vi "3D Shape Test Bench.vi"() -> ()   [LabVIEW 2017]
uses:
  <vilib>/picture/3D Picture Control/NI_3D Picture Control.lvlib
  <vilib>/robotics/Kinematics/NI_Kinematics.lvlib
  Controls/Room Dimensions.ctl
  <vilib>/userdefined/High Color/IMAQdx.ctl
  <vilib>/vision/Image Controls.llb/IMAQ Image.ctl
  <vilib>/vision/Avi.llb/IMAQ AVI2 Refnum.ctl
  Controls/Position.ctl
  Controls/Orientation.ctl
  Controls/Rigid Body Info.ctl
  Controls/Frame Grabber Data.ctl
  Controls/Dimensions.ctl
  Controls/Recording Settings.ctl
  Controls/Operator.ctl
  Controls/Operator Settings.ctl
  Controls/Refnums.ctl
  Controls/Patient Settings.ctl
panel:
  in  "Dimensions":T1={"Probe Dimensions"={"Probe Width"=0.0, "Probe Depth"=1.0, "Probe Height"=0.0}, "Room Dimensions"={"Room Width"=0.0, "Room Depth"=0.0, "Room Height"=0.0}}
  in  "Frame Grabber Data In":T3={"Camera Session"="", "Frame"="remote image 0000000019B07D24", "AVI Refnum"=refnum, "Codecs"=["Cinepak Codec by Radius", "Intel IYUV codec", "Microsoft Video 1", "FF Video Codec 1 (FFV1) (NI Vision)", "Motion JPEG (NI Vision)", "Y800 Uncompressed Grey Scale (NI Vision)", "YUV 4:2:0 Planar (NI Vision)"], "Frame number"=0, "Tracking File Refnum"=refnum, "Tick Count"=0, "Probe Object"=refnum, "Playback Probe Data"=[], "Rigid Body"={"Position"={"x (mm)"=0.0, "y (mm)"=0.0, "z (mm)"=0.0}, "Orientation"={"Pitch (rad)"=0.0, "Yaw (rad)"=0.0, "Roll (rad)"=0.0}, "Quaternion"={"qx"=0.0, "qy"=0.0, "qz"=0.0, "qw"=0.0}, "Tracked?"=FALSE}, "Total no frames playback"=0, "Video FPS"=0.0, "Camera connected?"=FALSE, "Scene"=refnum, "Cropped Frame"=refnum, "Tracker FPS"=0.0, "Crop ROI"=[], "Presentation Values"=[], "Elapsed time (ms)"=0, "Camera frames playback"=0, "Refnums"={"Live Refnum"=refnum, "Record Refnum"=refnum, "Playback Refnum"=refnum, "Frame Slider Refnum"=refnum, "Pause Refnum"=refnum, "Home Refnum"=refnum, "Set Crop Refnum"=refnum, "Clear Crop Refnum"=refnum, "stop refnum"=refnum, "Playback Rate Refnum"=refnum, "Presentation Refnum"=refnum, "Crop Time Frame Slider Refnum"=refnum, "Cancel Save Refnum"=refnum, "Reverse Playback Refnum"=refnum, "Recording Settings Refnum"=refnum, "Continuous Playback Refnum"=refnum, "Annotation Refnum"=refnum, "Export All Refnum"=refnum, "Export List Refnum"=refnum, "Fill List Refnum"=refnum, "Save Crop Refnum"=refnum, "Skip Forward Refnum"=refnum, "Skip Backward Refnum"=refnum, "Single Annotation Refnum"=refnum, "Load Video Refnum"=refnum, "Set Start Refnum"=refnum, "Set End Refnum"=refnum, "Add to List Refnum"=refnum, "List of Annotations Refnum"=refnum, "Camera Frame Refnum"=refnum, "Load Image Refnum"=refnum, "Saving Refnum"=refnum}, "Dimensions"={"Probe Dimensions"={"Probe Width"=0.0, "Probe Depth"=1.0, "Probe Height"=0.0}, "Room Dimensions"={"Room Width"=0.0, "Room Depth"=0.0, "Room Height"=0.0}}, "Playback Data As Strings"=[], "Cropped Tracking File Refnum"=refnum, "Cropped AVI Refnum"=refnum, "Header"=[], "Total euclidian distance"=0.0}
  out "Error Out":errorcluster={"status"=TRUE, "code"=1088, "source"="Property Node (arg 2) in NI_3D Picture Control.lvlib:Create Box.vi->Create 3D Shapes.vi->3D Shape Test Bench.vi"}
  in  "Error In":errorcluster
  in  "Initial Probe Position":cluster{"X":sgl, "Y":sgl, "Z":sgl}
  in  "Orientation":cluster{"X":sgl, "Y":sgl, "Z":sgl}
  in  "Stop Button":bool
  out "Scene":refnum<vi>(3d-picture)
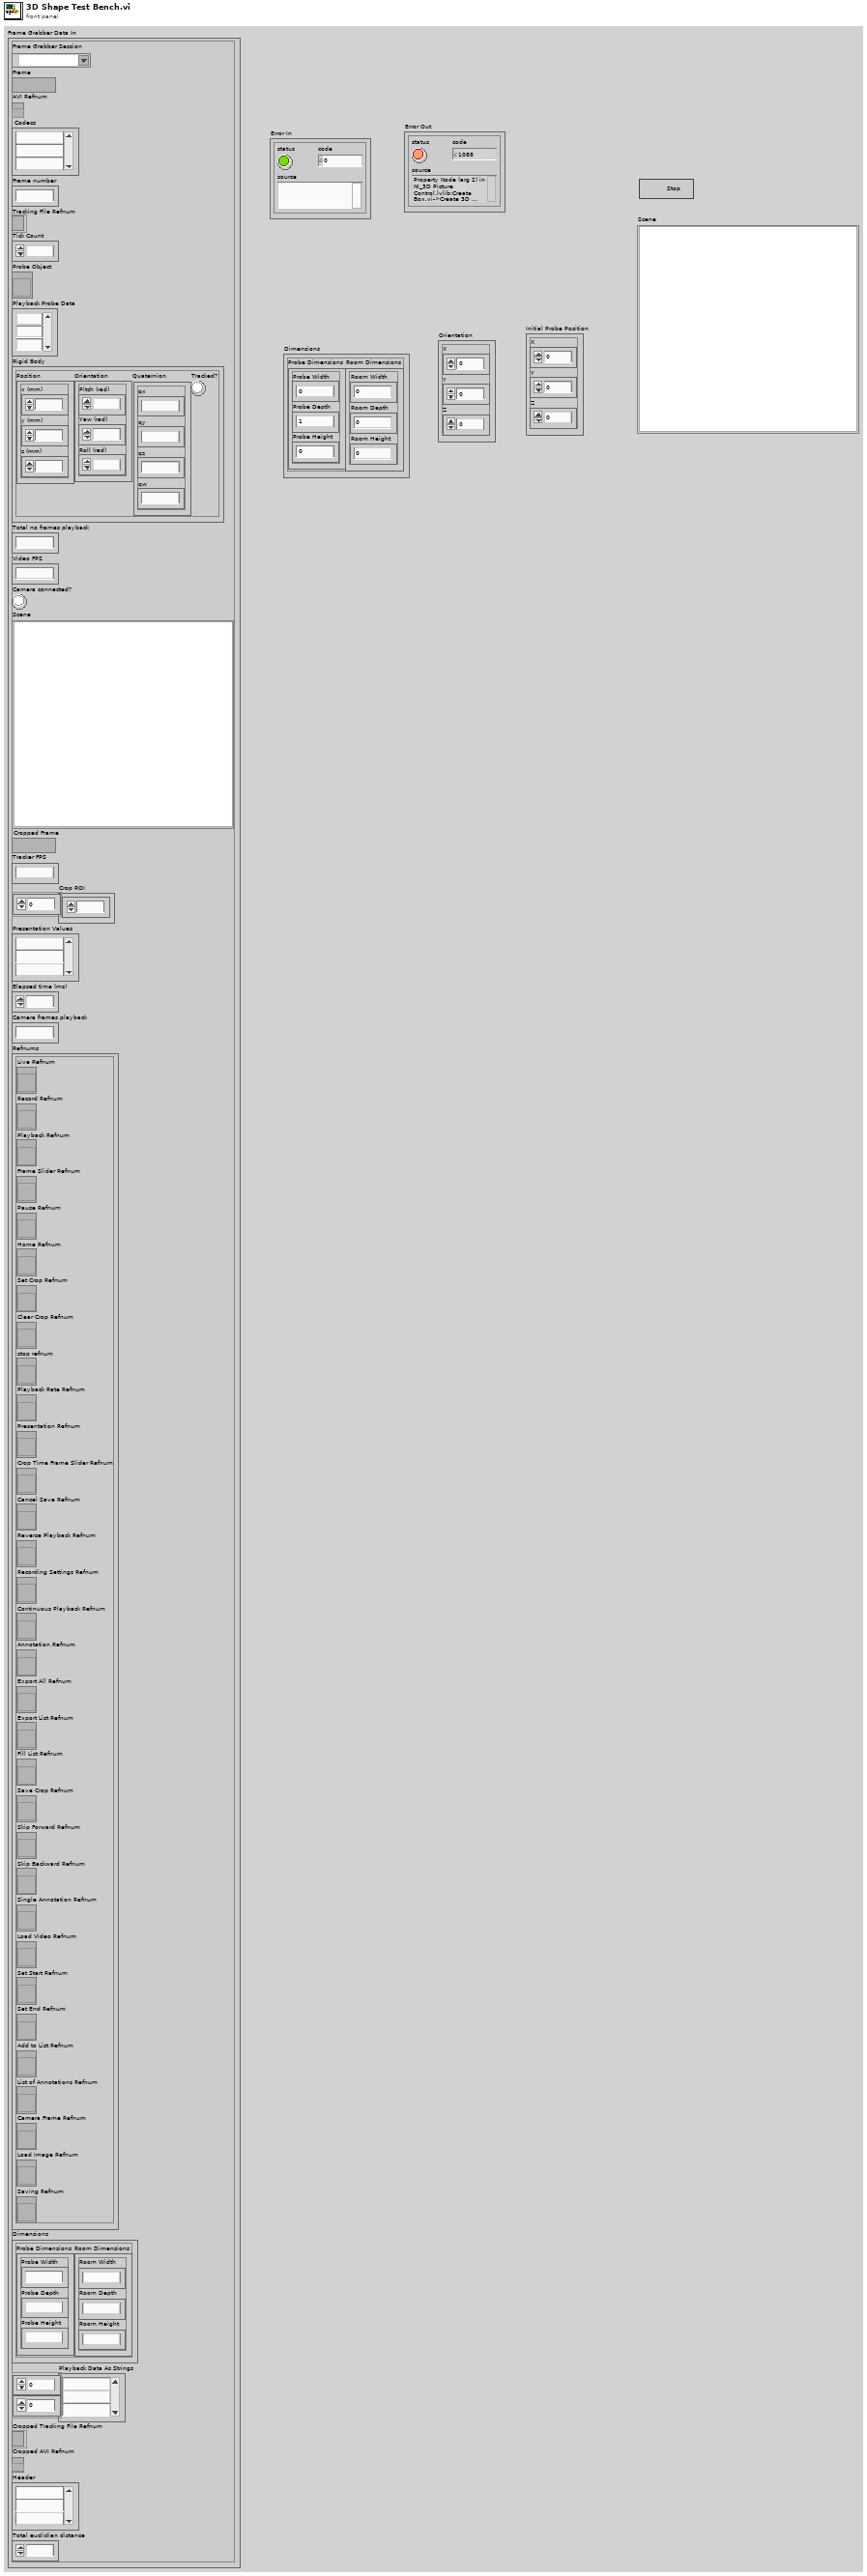
[diagram p1: front panel]
types:
  T1 = typedef "Dimensions.ctl" = cluster{"Probe Dimensions":cluster{"Probe Width":sgl, "Probe Depth":sgl, "Probe Height":sgl}, "Room Dimensions":T2}
  T2 = typedef "Room Dimensions.ctl" = cluster{"Room Width":dbl, "Room Depth":dbl, "Room Height":dbl}
  T3 = typedef "Frame Grabber Data.ctl" = cluster{"Camera Session":T4, "Frame":T5, "AVI Refnum":T6, "Codecs":string[], "Frame number":u32, "Tracking File Refnum":refnum<file>, "Tick Count":u32, "Probe Object":refnum<vi>, "Playback Probe Data":dbl[][], "Rigid Body":T7, "Total no frames playback":i32, "Video FPS":dbl, "Camera connected?":bool, "Scene":refnum<vi>, "Cropped Frame":T5, "Tracker FPS":dbl, "Crop ROI":i32[], "Presentation Values":string[], "Elapsed time (ms)":u32, "Camera frames playback":u32, "Refnums":T10, "Dimensions":T1, "Playback Data As Strings":string[][], "Cropped Tracking File Refnum":refnum<file>, "Cropped AVI Refnum":T6, "Header":string[], "Total euclidian distance":dbl}
  T4 = typedef "IMAQdx.ctl" = refnum<k21>
  T5 = typedef "IMAQ Image.ctl" = refnum<image>
  T6 = typedef "IMAQ AVI2 Refnum.ctl" = refnum<k20>
  T7 = typedef "Rigid Body Info.ctl" = cluster{"Position":T8, "Orientation":T9, "Quaternion":cluster{"qx":sgl, "qy":sgl, "qz":sgl, "qw":sgl}, "Tracked?":bool}
  T8 = typedef "Position.ctl" = cluster{"x (mm)":sgl, "y (mm)":sgl, "z (mm)":sgl}
  T9 = typedef "Orientation.ctl" = cluster{"Pitch (rad)":sgl, "Yaw (rad)":sgl, "Roll (rad)":sgl}
  T10 = typedef "Refnums.ctl" = cluster{"Live Refnum":refnum<vi>, "Record Refnum":refnum<vi>, "Playback Refnum":refnum<vi>, "Frame Slider Refnum":refnum<vi>, "Pause Refnum":refnum<vi>, "Home Refnum":refnum<vi>, "Set Crop Refnum":refnum<vi>, "Clear Crop Refnum":refnum<vi>, "stop refnum":refnum<vi>, "Playback Rate Refnum":refnum<vi>, "Presentation Refnum":refnum<vi>, "Crop Time Frame Slider Refnum":refnum<vi>, "Cancel Save Refnum":refnum<vi>, "Reverse Playback Refnum":refnum<vi>, "Recording Settings Refnum":refnum<vi>, "Continuous Playback Refnum":refnum<vi>, "Annotation Refnum":refnum<vi>, "Export All Refnum":refnum<vi>, "Export List Refnum":refnum<vi>, "Fill List Refnum":refnum<vi>, "Save Crop Refnum":refnum<vi>, "Skip Forward Refnum":refnum<vi>, "Skip Backward Refnum":refnum<vi>, "Single Annotation Refnum":refnum<vi>, "Load Video Refnum":refnum<vi>, "Set Start Refnum":refnum<vi>, "Set End Refnum":refnum<vi>, "Add to List Refnum":refnum<vi>, "List of Annotations Refnum":refnum<vi>, "Camera Frame Refnum":refnum<vi>, "Load Image Refnum":refnum<vi>, "Saving Refnum":refnum<vi>}
  T11 = typedef "Frame Grabber Data.ctl" = cluster{"Camera Session":T4, "Frame":T5, "AVI Refnum":T6, "Codecs":string[], "Frame number":u32, "Tracking File Refnum":refnum<file>, "Tick Count":u32, "Probe Object":refnum<vi>, "Playback Probe Data":dbl[][], "Rigid Body":T7, "Total no frames playback":i32, "Video FPS":dbl, "Camera connected?":bool, "Scene":refnum<vi>, "Cropped Frame":T5, "Tracker FPS":dbl, "Crop ROI":i32[], "Presentation Values":string[], "Elapsed time (ms)":u32, "Camera frames playback":u32, "Refnums":T10, "Dimensions":T1, "Playback Data As Strings":string[][], "Cropped Tracking File Refnum":refnum<file>, "Cropped AVI Refnum":T6, "Header":string[], "Total euclidian distance":dbl, "Annotation File Path":path, "Playback File Path":path, "Size per frame":dbl, "Ground Truth File Refnum":refnum<file>, "Annotation Array":string[], "Annotation TIFFs Folder":path, "overwriting open file?":bool, "Image Sequence":T5[], "Video/Image Flag":T12, "Image sequence?":bool, "Image sequence filenames":string[], "Mask":T5, "Crop Type":T13}
  T12 = typedef "Crop Video State.ctl" = enum16{"Init", "Wait", "Load Image", "Load Video", "Play/Pause", "Playback Video Frame", "Display Image", "Save Image Sequence", "Save Video", "Export List", "Export All", "Close", "Set Crop Area", "Reset Crop Area", "Crop Inside", "Crop Outside", "Multi-Crop", "Re-Open Files", "Annotate Frame", "Annotate Clip", "Add to List", "Fill List", "Set Start", "Set End", "Error Handling", "Shutdown"}
  T13 = typedef "Crop Type.ctl" = enum16{"Rectangle", "Annulus"}
  T14 = typedef "NI_Matrix.lvlib/RealMatrix.ctl" = dbl[][]
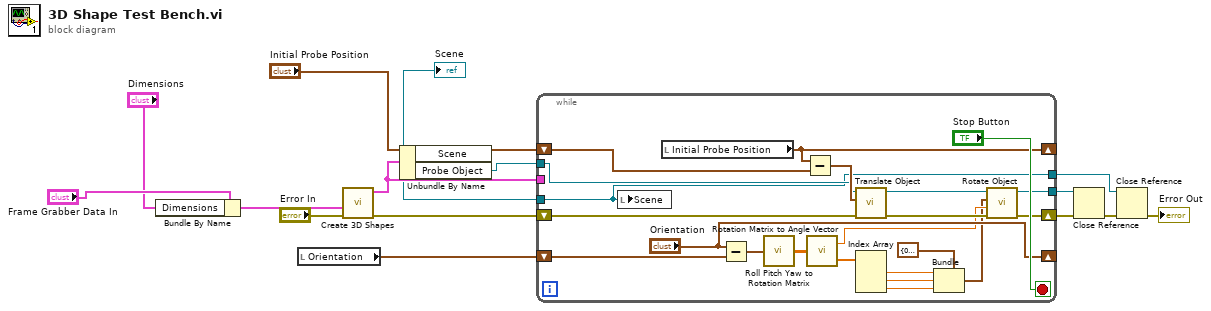
[diagram p0: block diagram]
diagram:
  n1 = Bundle By Name(cluster="Frame Grabber Data In", "Dimensions"="Dimensions") -> (w2:T3)
  n2 = local read "Orientation"() -> (w15:cluster{"X":sgl, "Y":sgl, "Z":sgl})
  n3 = call "Create 3D Shapes.vi"("error in (no error)"="Error In", "Frame Grabber Data In"=w2) -> ("error out"=w14:errorcluster, "Frame Grabber Data Out"=w7:T11)  [unwired: 8 in]
  n4 = Unbundle By Name(w7) -> ("Scene"=w6:refnum<vi>, "Probe Object"=w5:refnum<vi>)
  "Scene" <- w6
  n5 = while {
    shift-right: ["Orientation"] -> _
    shift-left: w15 -> [w33]
    shift-right: [w18] -> _
    shift-left: "Initial Probe Position" -> [w30]
    shift-right: [w34] -> w12
    shift-left: w14 -> [w36]
    tunnel: w7 -> [_]
    tunnel: [w31] -> w13
    tunnel: w6 -> [w16]
    tunnel: w5 -> [w17]
    tunnel: [w16] -> w4
    stop <- "Stop Button" stop-if-true
    n6 = local write "Scene"(w16) -> ()
    n7 = local read "Initial Probe Position"() -> (w18:cluster{"X":sgl, "Y":sgl, "Z":sgl})
    n8 = Subtract(x="Orientation", y=w33) -> (x-y=w25:cluster{"X":sgl, "Y":sgl, "Z":sgl})
    n9 = call <vilib>:"Roll Pitch Yaw to Rotation Matrix.vi"("angles"=w25) -> ("rotation matrix"=w27:T14)
    n10 = Subtract(x=w18, y=w30) -> (x-y=w29:cluster{"X":sgl, "Y":sgl, "Z":sgl})
    n11 = call <vilib>:"Rotation Matrix to Angle Vector.vi"("rotation matrix"=w27) -> ("angle"=w26:dbl, "vector"=w23:dbl[])
    n12 = call <vilib>:"Translate Object.vi"("error in (no error)"=w36, "Translation"=w29, "Scene.Object In"=w17) -> ("error out"=w35:errorcluster, "Scene.Object Out"=w32:refnum<vi>)  [unwired: 7 in]
    n13 = Index Array(array=w23) -> (element #1=w20:dbl, element #2=w21:dbl, element #3=w22:dbl)  [unwired: 3 in]
    n14 = Bundle(cluster=cluster{"X":sgl, "Y":sgl, "Z":sgl} {"X"=0.0, "Y"=0.0, "Z"=0.0} ("Axis"), "X"=w20, "Y"=w21, "Z"=w22) -> (w19:cluster{"X":sgl, "Y":sgl, "Z":sgl})
    n15 = call <vilib>:"Rotate Object.vi"("error in (no error)"=w35, "Angle"=w26, "Axis"=w19, "Scene.Object In"=w32) -> ("error out"=w34:errorcluster, "Scene.Object Out"=w31:refnum<vi>)  [unwired: 6 in]
  }
  n16 = Close Reference(reference=w13, error in (no error)=w12) -> (error out=w11:errorcluster)
  n17 = Close Reference(reference=w4, error in (no error)=w11) -> (error out=→"Error Out":errorcluster)
